vi "cno_find initial solution.vi"(0 "P0":dbl[](array[numeric]), 1 "cno data":T1, 5 "A":dbl[][](array[numeric]), 7 "B":dbl[](array[numeric]), 9 "CONSTRAINT":dbl[](array[numeric]), 11 "error":errorcluster, 12 "PB":dbl[][](array[numeric])) -> (2 "cno data":T1, 4 "P0":dbl[](array[numeric]), 6 "A":dbl[][](array[numeric]), 8 "B":dbl[](array[numeric]), 15 "error":errorcluster)   [LabVIEW 2020, in "NI_Gmath.lvlib"]
uses:
  <vilib>/gmath/NI_Gmath.lvlib
  <vilib>/gmath/NumericalOptimization/cno_data.ctl
  <vilib>/Analysis/baseanly.llb/Real A x B.vi
  <vilib>/Analysis/baseanly.llb/A x Vector.vi
  <vilib>/gmath/NumericalOptimization/Matrix left divisionMV.vi
  <vilib>/gmath/NumericalOptimization/ones_1d.vi
  <vilib>/gmath/NumericalOptimization/zeroes_1d.vi
  <vilib>/Analysis/7linalg.llb/Create Special Real Matrix.vi
  <vilib>/Analysis/NI_AALBase.lvlib
  <vilib>/Analysis/NI_AALPro.lvlib
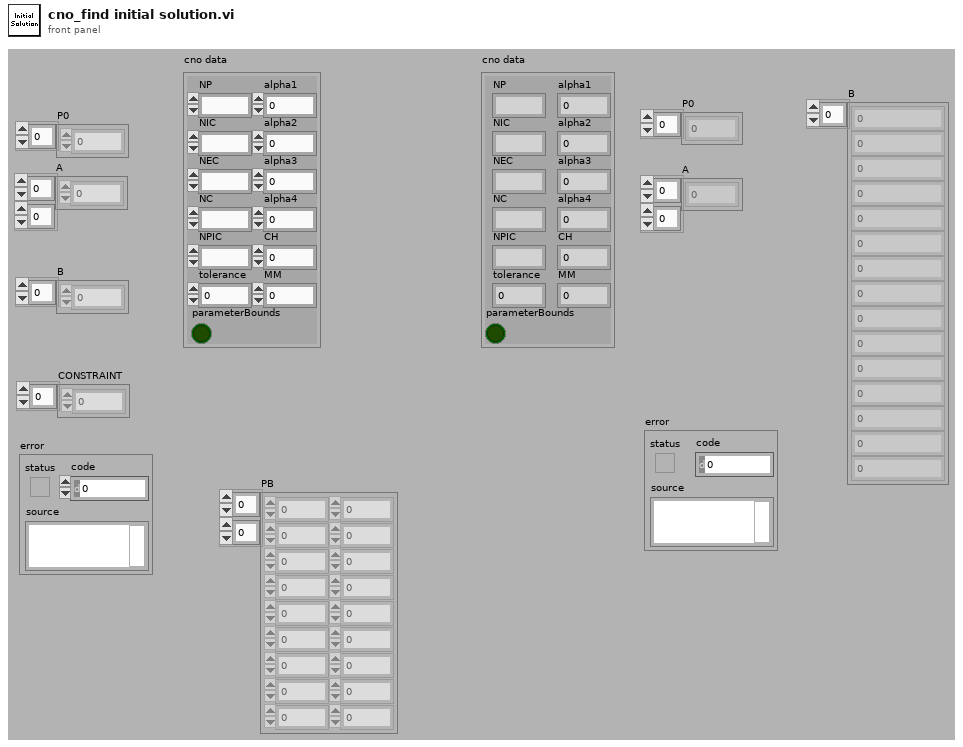
[diagram p1: front panel]
types:
  T1 = typedef "NI_Gmath.lvlib/cno_data.ctl" = cluster{"NP":i32, "NIC":i32, "NEC":i32, "NC":i32, "NPIC":i32, "parameterBounds":bool, "alpha1":dbl, "alpha2":dbl, "alpha3":dbl, "alpha4":dbl, "CH":i32, "MM":i32, "tolerance":dbl}
  T2 = enum32{"Identity", "Diagonal", "Toepliz", "Vandermonde", "Companion"}
  T3 = typedef "NI_Matrix.lvlib/RealMatrix.ctl" = dbl[][]
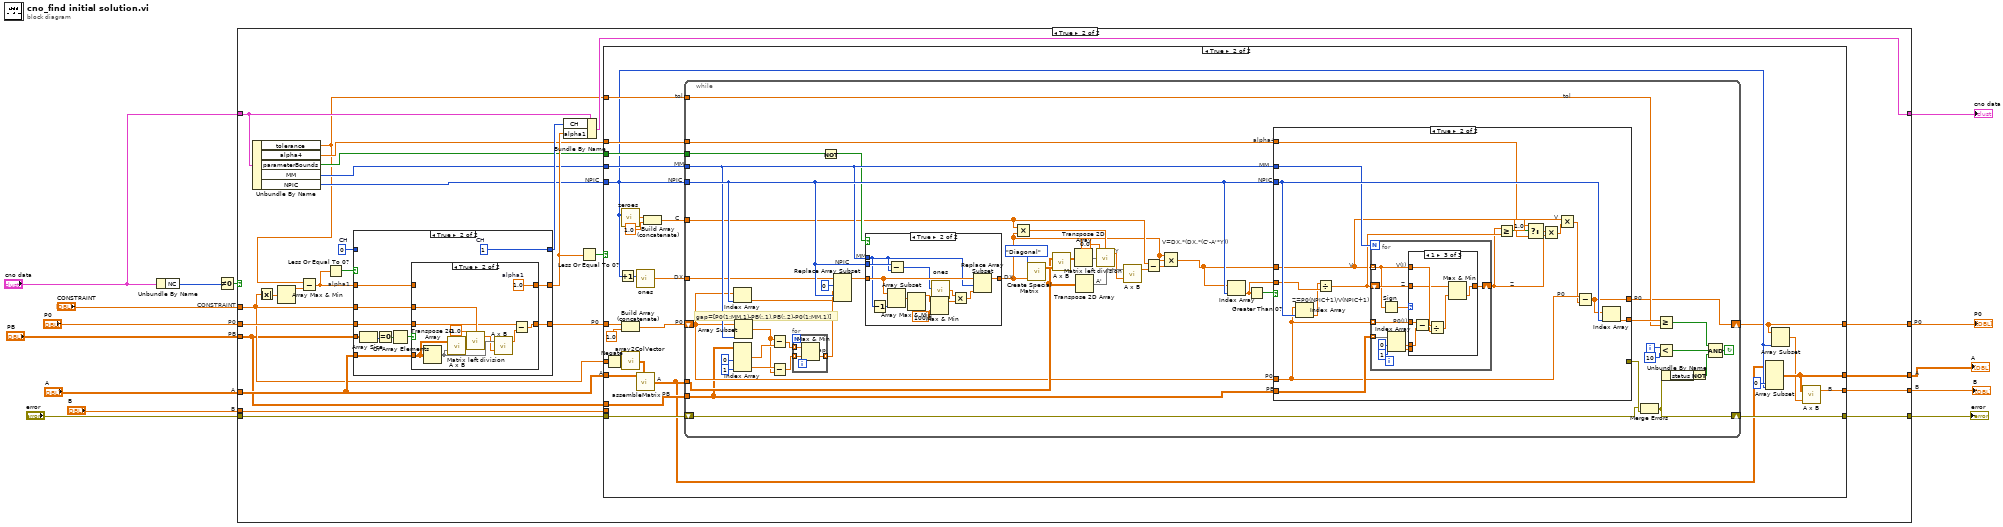
[diagram p0: block diagram]
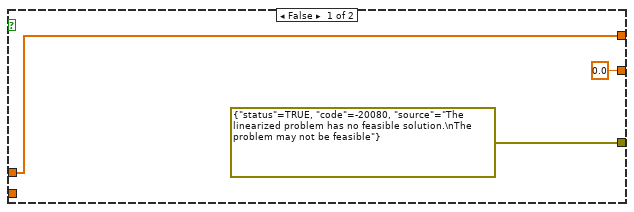
[diagram p4: hidden frame]
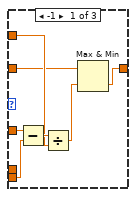
[diagram p5: hidden frame]
diagram:
  # "B"
  # "A"
  # "B"
  # "P0"
  # "PB"
  # "A"
  # "P0"
  # "CONSTRAINT"
  n1 = Unbundle By Name("cno data") -> ("NC"=w5:i32)
  n2 = Not Equal To 0?(x=w5) -> (x != 0?=w6:bool)
  n3 = case shown="True" w6 {
    tunnel: "CONSTRAINT" -> [_ w36]
    tunnel: "PB" -> [_ w35]
    tunnel: "P0" -> [w19 w41]
    tunnel: "A" -> [w18 w37]
    tunnel: [w19 w31] -> w11
    tunnel: "error" -> [w17 w34]
    tunnel: [w17 w33] -> w14
    tunnel: [w18 w32] -> w13
    tunnel: "cno data" -> [w16 w25]
    tunnel: [w15 w28] -> w12
    tunnel: [w16 w27] -> w1
    tunnel: "B" -> [w15 w26]
    frame False {
    }
    frame True {
      w42 = 0  # CH
      # "A"
      # "NPIC"
      # "P0"
      # "alpha1"
      n4 = Unbundle By Name(w25) -> ("tolerance"=w20:dbl, "alpha4"=w24:dbl, "parameterBounds"=w23:bool, "MM"=w21:i32, "NPIC"=w22:i32)
      n5 = Absolute Value(x=w36) -> (abs(x)=w45:dbl[])
      n6 = Array Max & Min(array=w45) -> (max value=w44:dbl)  [unwired: 3 out]
      n7 = Subtract(x=w20, y=w44) -> (x-y=w40:dbl)
      n8 = Less Or Equal To 0?(x=w40) -> (x <= 0?=w43:bool)
      n9 = case shown="True" w43 {
        tunnel: w42 -> [w187 _]
        tunnel: [w187 w198] -> w30
        tunnel: w35 -> [_ w195]
        tunnel: w41 -> [w185 w193]
        tunnel: w37 -> [_ w192]
        tunnel: w36 -> [_ w191]
        tunnel: w40 -> [w186 w190]
        tunnel: [w186 w189] -> w29
        tunnel: [w185 w188] -> w38
        frame False {
        }
        frame True {
          w198 = 1  # CH
          n10 = Array Size(array=w195) -> (size(s)=w196:i32[])
          n11 = Equal To 0?(x=w196) -> (x = 0?=w197:bool[])
          n12 = Or Array Elements(Boolean array=w197) -> (logical OR=w194:bool)
          n13 = case shown="True" w194 {
            tunnel: w193 -> [w200 w205]
            tunnel: w192 -> [_ w210]
            tunnel: w191 -> [_ w208]
            tunnel: [w200 w203] -> w188
            tunnel: w190 -> [w199 _]
            tunnel: [w199 w202] -> w189
            frame False {
            }
            frame True {
              w202 = 1.0  # alpha1
              n14 = Transpose 2D Array(2D array=w210) -> (transposed array=w207:dbl[][])
              n15 = call-poly <vilib>:"A x B.vi"("B"=w207, "A"=w210) -> ("A x B"=w209:T3)  [unwired: 1 out]
              n16 = call-poly <vilib>:"Matrix left division.vi"("A"=w208, "B"=w209, "SVD relative tolerance"=-1.0) -> ("B\\A"=w206:dbl[])  [unwired: 1 in, 1 out]
              n17 = call-poly <vilib>:"A x B.vi"("Vector"=w206, "A"=w207) -> ("A x Vector"=w204:dbl[])  [unwired: 1 out]
              n18 = Subtract(x=w205, y=w204) -> (x-y=w203:dbl[])
            }
          }
        }
      }
      n19 = Bundle By Name(cluster=w25, "CH"=w30, "alpha1"=w29) -> (w27:T1)
      n20 = Less Or Equal To 0?(x=w29) -> (x <= 0?=w39:bool)
      n21 = case shown="True" w39 {
        tunnel: w38 -> [w48 w75]
        tunnel: w22 -> [_ w57]
        tunnel: w37 -> [w49 w74]
        tunnel: w36 -> [_ w73]
        tunnel: w21 -> [_ w68]
        tunnel: w35 -> [_ w64]
        tunnel: w23 -> [_ w63]
        tunnel: w24 -> [_ w62]
        tunnel: w20 -> [_ w61]
        tunnel: w34 -> [w47 w60]
        tunnel: [w47 w59] -> w33
        tunnel: [w49 w56] -> w32
        tunnel: [w48 w55] -> w31
        tunnel: [w46 w54] -> w28
        tunnel: w26 -> [w46 _]
        frame False {
        }
        frame True {
          # "B"
          # "NPIC"
          # "PB"
          # "DX"
          # "C"
          # "MM"
          # "tol"
          # "P0"
          # "A"
          n22 = Negate(x=w73) -> (-x=w53:dbl[])
          n23 = Increment(x=w57) -> (x+1=w69:i32)
          n24 = call-poly <vilib>:"zeroes.vi"("m"=w57) -> ("ones"=w71:dbl[])  [unwired: 7 in]
          n25 = Build Array (concatenate)(w75, 1.0 ("new element/subarray")) -> (w67:dbl[])
          n26 = call <vilib>:"array2ColVector.vi"("vector"=w53) -> ("col vector"=w72:dbl[][])
          n27 = call-poly <vilib>:"ones.vi"("m"=w69) -> ("ones"=w65:dbl[])  [unwired: 7 in]
          n28 = call <vilib>:"assembleMatrix.vi"("A"=w74, "B"=w72) -> ("ABCD"=w51:dbl[][])  [unwired: 3 in]
          n29 = Build Array (concatenate)(w71, 1.0) -> (w66:dbl[])
          n30 = while {
            tunnel: w68 -> [w122]
            tunnel: w51 -> [w105]
            tunnel: w66 -> [w102]
            tunnel: w65 -> [w107]
            tunnel: w64 -> [w94]
            tunnel: w57 -> [w123]
            tunnel: w63 -> [w113]
            tunnel: w62 -> [w93]
            shift-right: [w88] -> w59
            shift-left: w60 -> [w91]
            shift-right: [w78] -> w55
            shift-left: w67 -> [w97]
            tunnel: w61 -> [w86]
            i -> [w85]
            stop <- w79 continue-if-true
            # "NPIC"
            # "MM"
            # "P0"
            # "alpha4"
            # "tol"
            # "PB"
            # "MM"
            # "NPIC"
            # "P0"
            # "V=DX.*(DX.*(C'-A'*Y))"
            # "A'"
            # "Y"
            # "DX"
            # "gap"
            # "gap=[P0(1:MM,1)-PB(:,1),PB(:,2)-P0(1:MM,1)]"
            n31 = Index Array(array=w97, index=w123) -> (element=w114:dbl)
            n32 = Index Array(array=w94, index (col) #1=0 ("disabled index (col)"), index (col) #2=1 ("index (col)")) -> (element #1=w119:dbl[], element #2=w118:dbl[])  [unwired: 2 in]
            n33 = Array Subset(array=w97, length=w122) -> (w117:dbl[])  [unwired: 1 in]
            n34 = Subtract(x=w117, y=w119) -> (x-y=w90:dbl[])
            n35 = Subtract(x=w118, y=w117) -> (x-y=w89:dbl[])
            n36 = for {
              tunnel: w90 -> [w184] mode=indexing
              tunnel: w89 -> [w183] mode=indexing
              tunnel: [w182] -> w116 mode=indexing
              n37 = Max & Min(x=w184, y=w183) -> (min(x,y)=w182:dbl)  [unwired: 1 out]
            }
            n38 = Not(x=w113) -> (.not. x?=w111:bool)
            n39 = Replace Array Subset(array=w107, new element #1=w116, index #1=0 ("index"), new element #2=w114, index #2=w123) -> (w112:dbl[])
            n40 = case shown="True" w111 {
              tunnel: w112 -> [w169 w181]
              tunnel: w122 -> [_ w173]
              tunnel: w123 -> [_ w174]
              tunnel: [w169 w170] -> w77
              frame False {
              }
              frame True {
                n41 = Decrement(x=w173) -> (x-1=w180:i32)
                n42 = Array Subset(array=w181, length=w180) -> (w179:dbl[])  [unwired: 1 in]
                n43 = Subtract(x=w174, y=w173) -> (x-y=w172:i32)
                n44 = Array Max & Min(array=w179) -> (max value=w178:dbl)  [unwired: 3 out]
                n45 = Max & Min(x=w178, y=100.0) -> (max(x,y)=w176:dbl)  [unwired: 1 out]
                n46 = call-poly <vilib>:"ones.vi"("m"=w172) -> ("ones"=w175:dbl[])  [unwired: 7 in]
                n47 = Multiply(x=w175, y=w176) -> (x*y=w171:dbl[])
                n48 = Replace Array Subset(array=w181, new element=w171, index=w173) -> (w170:dbl[])
              }
            }
            n49 = Multiply(x=w102, y=w77) -> (x*y=w106:dbl[])
            n50 = call-poly <vilib>:"Create Special Matrix.vi"("matrix type"=T2."Diagonal", "Input Vector1"=w77) -> ("Special Matrix"=w110:T3)  [unwired: 3 in, 1 out]
            n51 = call-poly <vilib>:"A x B.vi"("B"=w110, "A"=w105) -> ("A x B"=w109:T3)  [unwired: 1 out]
            n52 = Transpose 2D Array(2D array=w109) -> (transposed array=w108:T3)
            n53 = Transpose 2D Array(2D array=w105) -> (transposed array=w104:dbl[][])
            n54 = call-poly <vilib>:"Matrix left division.vi"("A"=w106, "B"=w108, "SVD relative tolerance"=0.0) -> ("B\\A"=w103:dbl[])  [unwired: 1 in, 1 out]
            n55 = call-poly <vilib>:"A x B.vi"("Vector"=w103, "A"=w104) -> ("A x Vector"=w101:dbl[])  [unwired: 1 out]
            n56 = Subtract(x=w102, y=w101) -> (x-y=w99:dbl[])
            n57 = Compound Arithmetic op=MULTIPLY(w77, w77, w99) -> (w95:dbl[])
            n58 = Index Array(array=w95, index=w123) -> (element=w96:dbl)
            n59 = Greater Than 0?(x=w96) -> (x > 0?=w98:bool)
            n60 = case shown="True" w98 {
              tunnel: w97 -> [w125 w138]
              tunnel: w123 -> [_ w143]
              tunnel: w96 -> [_ w128]
              tunnel: w122 -> [_ w141]
              tunnel: w95 -> [_ w132]
              tunnel: w94 -> [_ w140]
              tunnel: w93 -> [_ w142]
              tunnel: [w125 w130] -> w78
              tunnel: [0.0 w129] -> w87
              tunnel: [errorcluster {"status"=TRUE, "code"=-20080, "source"="The linearized problem has no feasible solution.\nThe problem may not be feasible"} ("error") _] -> w92
              frame False {
              }
              frame True {
                # "V"
                # "P0"
                # "V"
                # "Z"
                # "Z=P0(NPIC+1)/V(NPIC+1)"
                n61 = Index Array(array=w138, index=w143) -> (element=w127:dbl)
                n62 = Divide(x=w127, y=w128) -> (x/y=w139:dbl)
                n63 = for {
                  N: w141 -> [_]
                  tunnel: w132 -> [w145] mode=indexing
                  tunnel: w140 -> [w152] mode=indexing
                  tunnel: w138 -> [w146] mode=indexing
                  shift-right: [w144] -> w133
                  shift-left: w139 -> [w150]
                  # "V(I)"
                  # "P0(I)"
                  # "Z"
                  n64 = Sign(1:w145) -> (0:w153:dbl)
                  n65 = Index Array(array=w152, index #1=0 ("index"), index #2=1 ("index")) -> (element #1=w148:dbl, element #2=w147:dbl)
                  n66 = case shown="1" w153 {
                    tunnel: w150 -> [w158 w161 w166]
                    tunnel: w148 -> [_ _ w162]
                    tunnel: w147 -> [w154 _ _]
                    tunnel: w146 -> [w155 _ w163]
                    tunnel: w145 -> [w159 _ w167]
                    tunnel: [w156 w161 w164] -> w144
                    frame -1 {
                      n67 = Subtract(x=w155, y=w154) -> (x-y=w160:dbl)
                      n68 = Divide(x=w160, y=w159) -> (x/y=w157:dbl)
                      n69 = Max & Min(x=w158, y=w157) -> (min(x,y)=w156:dbl)  [unwired: 1 out]
                    }
                    frame 0, Default {
                    }
                    frame 1 {
                      n70 = Subtract(x=w163, y=w162) -> (x-y=w168:dbl)
                      n71 = Divide(x=w168, y=w167) -> (x/y=w165:dbl)
                      n72 = Max & Min(x=w166, y=w165) -> (min(x,y)=w164:dbl)  [unwired: 1 out]
                    }
                  }
                }
                n73 = Greater Or Equal?(x=w133, y=w139) -> (x >= y?=w136:bool)
                n74 = Select(t=1.0, s=w136, f=w142) -> (s? t:f=w134:dbl)
                n75 = Multiply(x=w134, y=w133) -> (x*y=w131:dbl)
                n76 = Multiply(x=w132, y=w131) -> (x*y=w137:dbl[])
                n77 = Subtract(x=w138, y=w137) -> (x-y=w130:dbl[])
                n78 = Index Array(array=w130, index=w143) -> (element=w129:dbl)
              }
            }
            n79 = Merge Errors(w91, w92) -> (w88:errorcluster)
            n80 = Greater Or Equal?(x=w87, y=w86) -> (x >= y?=w82:bool)
            n81 = Less?(x=w85, y=10) -> (x < y?=w81:bool)
            n82 = Unbundle By Name(w88) -> ("status"=w83:bool)
            n83 = Not(x=w83) -> (.not. x?=w80:bool)
            n84 = Compound Arithmetic op=AND(w82, w81, w80) -> (w79:bool)
          }
          n85 = Array Subset(array=w51, index (col)=0 ("index"), length (col)=w57) -> (w56:dbl[][])  [unwired: 2 in]
          n86 = Array Subset(array=w55, length=w57) -> (w50:dbl[])  [unwired: 1 in]
          n87 = call-poly <vilib>:"A x B.vi"("Vector"=w50, "A"=w56) -> ("A x Vector"=w54:dbl[])  [unwired: 1 out]
        }
      }
    }
  }
  "error" <- w14
  "A" <- w13
  "B" <- w12
  "P0" <- w11
  "cno data" <- w1
